vi "RD Analog Out Node Phase Set.vi"(7 "degreePhase":dbl, 8 "error in (no error)":errorcluster caption="错误输入（无错误）", 9 "node":i32, 10 "ch":i32, 11 "handle":u64) -> (0 "error out":errorcluster caption="错误输出", 2 "function return":i32, 3 "handle out":u64)   [LabVIEW 2018, in "InstrumentsPlayground.lvlib"]
doc: "CLIFFAPI int CliffAnalogOutNodePhaseSet(FT_HANDLE handle,int ch,CLIFFAnalogOutNode node,double degreePhase);\nch: 0 ch1; 1 ch2;\nnode: Carrier = 0;FM = 1;AM = 2;\ndegreePhase: 0~360°"
uses:
  InstrumentsPlayground.lvlib
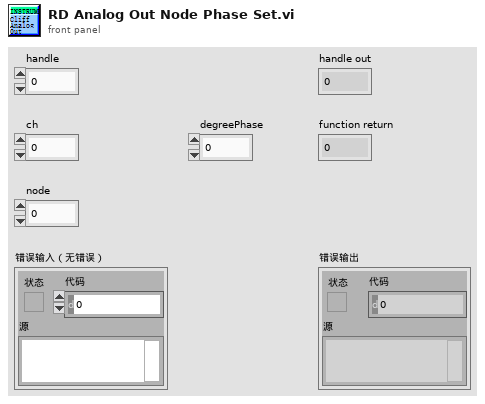
[diagram p1: front panel]
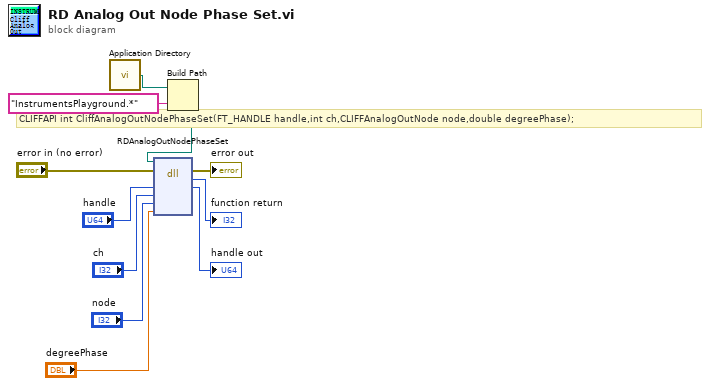
[diagram p0: block diagram]
diagram:
  # "CLIFFAPI int CliffAnalogOutNodePhaseSet(FT_HANDLE handle,int ch,CLIFFAnalogOutNode node,double degreePhase);"
  n1 = call <vilib>:"Application Directory.vi"() -> ("Application Directory"=w2:path)
  n2 = Build Path(base path=w2, name or relative path="InstrumentsPlayground.*" ("名称或相对路径")) -> (appended path=w1:path)
  n3 = dll-call lib="E:/work/YZCourse_Xtext/Cliff/API/LabVIEW lib/InstrumentsPlayground.*" fn="RDAnalogOutNodePhaseSet"(path in=w1, error in="error in (no error)", "handle"="handle", "ch"="ch", "node"="node", "degreePhase"="degreePhase") -> (error out=→"error out":errorcluster, "返回类型"=→"function return":i32, "handle"=→"handle out":u64)  [unwired: 4 in, 1 out]
